vi "TCL Select Fragments Nfrags1criterium.vi"(0 "event file":path, 1 "fragments":string[](array[string]), 3 "primary key":string, 4 "criterium":T1={"fragment"="", "values"=[], "operator"="is equal to"}, 5 "error in (no error)":errorcluster) -> (6 "fragments out":string[](array[string]), 7 "matches":string[][](array[string]), 8 "error out":errorcluster)   [LabVIEW 2010]
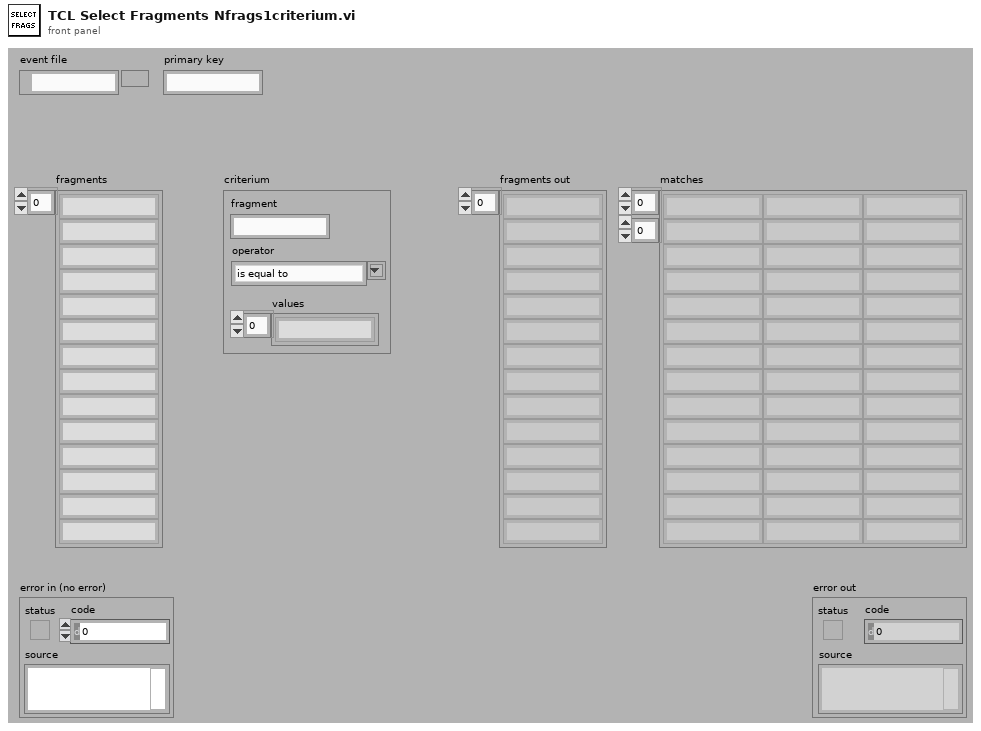
[diagram p1: front panel]
types:
  T1 = cluster{"fragment":string, "values":string[], "operator":string}
  T2 = cluster{"fragment":string, "values":string[], "operator":string}[]
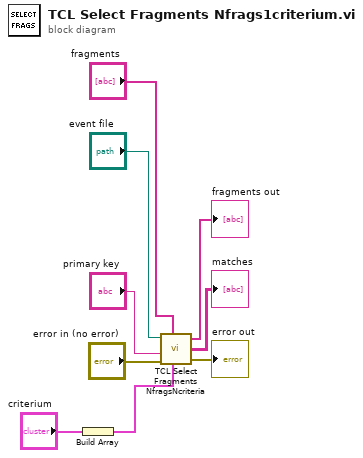
[diagram p0: block diagram]
diagram:
  n1 = Build Array("criterium") -> (w6:T2)
  n2 = call "TCL Select Fragments NfragsNcriteria.vi"("event file"="event file", "fragments"="fragments", "primary key"="primary key", "criteria"=w6, "error in (no error)"="error in (no error)") -> ("fragments out"=→"fragments out":string[], "matches"=→"matches":string[][], "error out"=→"error out":errorcluster)  [unwired: 1 in]
